vi "SETMODdll.vi"(8 "error in (no error)":errorcluster, 11 "Inputs":T2) -> (0 "error out":errorcluster, 3 "Outputs":T1)   [LabVIEW 2021]
doc: "subroutine SETMODdll(ncomp, htype, hmix, hcomp2, ierr, herr, htype_length, hmix_length, hcomp2_length, herr_length)\n\nSet model(s) other than the NIST-recommended (‘NBS’) ones.\n\nThis subroutine must be called before SETUP; it need not be called at all if the default (NIST-recommended)\nmodels are desired.\n\nINPUTS:\nncomp -- Number of components (1 for pure fluid) (integer)\nhtype -- Flag indicating which model to set (character*3)\n 'EOS': equation of state for thermodynamic properties\n 'ETA': viscosity\n 'TCX': thermal conductivity\n 'STN': surface tension\n 'NBS': reset all of the above model types and all subsidiary component models to 'NBS', values of hmix and hcomp are ignored.\nhmix -- Mixture model for the property specified in htype (character*3)\n Ignored if number of components = 1 \n Examples for hmix: \n ‘NBS’: use NIST recommendation for specified fluid/mixture \n ‘HMX’: mixture Helmholtz model for thermodynamic properties\n ‘ECS’: extended corresponding states for viscosity or therm. cond. \n ‘STX’: surface tension mixture model\nhcomp2 -- component model(s) to use for property specified in htype [array (1..ncomp) of character*3]\n 'NBS': NIST recommendation for specified fluid/mixture some allowable choices for an equation of state:\n 'FEQ': Helmholtz free energy model\n 'BWR': pure fluid modified Benedict-Webb-Rubin (MBWR)\n 'ECS': pure fluid thermo extended corresponding states some allowable choices for viscosity:\n 'ECS': extended corresponding states (all fluids)\n 'VS1': the 'composite' model for R134a, R152a, NH3, etc.\n 'VS2': Younglove-Ely model for hydrocarbons\n 'VS4': Generalized friction theory of Quinones-Cisneros and Deiters\n 'VS5': Chung et al. (1988) predictive model some allowable choices for thermal conductivity:\n 'ECS': extended corresponding states (all fluids)\n 'TC1': the 'composite' model for R134a, R152a, etc.\n 'TC2': Younglove-Ely model for hydrocarbons\n 'TC5': Chung et al. (1988) predictive model some allowable choices for surface tension:\n 'ST1': surface tension as f(tau); tau = 1 - T/Tc\n\nOUTPUTS:\nierr -- Error flag: 0 - Successful \n 113 - ncomp outside of bounds\nherr -- Error string (character*255)\nhtype_length -- length of variable htype (default: 3)\nhmix_length -- length of variable hmix (default: 3)\nhcomp2_length -- length of variable hcomp2 (default: 60)\nherr_length -- length of variable herr (default: 255)"
uses:
  REFPROP.dll
panel:
  # "REFPROP-SETMODdll.vi"
  # "void  SETMODdll(int32_t *ncomp, CStr htype, CStr hmix, CStr hcomp2, int32_t *ierr, CStr herr, int32_t htype_length, int32_t hmix_length, int32_t hcomp2_length, int32_t herr_length)"
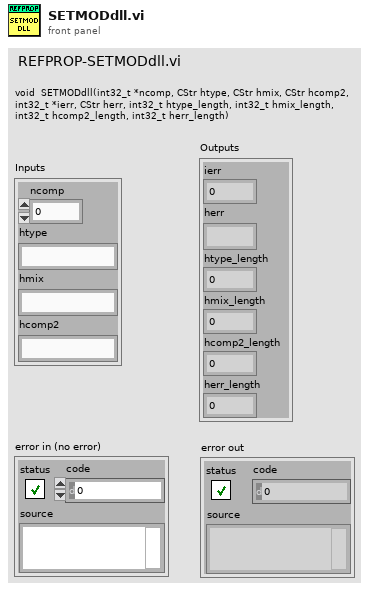
[diagram p1: front panel]
types:
  T1 = cluster{"ierr":i32, "herr":string, "htype_length":i32, "hmix_length":i32, "hcomp2_length":i32, "herr_length":i32}
  T2 = cluster{"ncomp":i32, "htype":string, "hmix":string, "hcomp2":string}
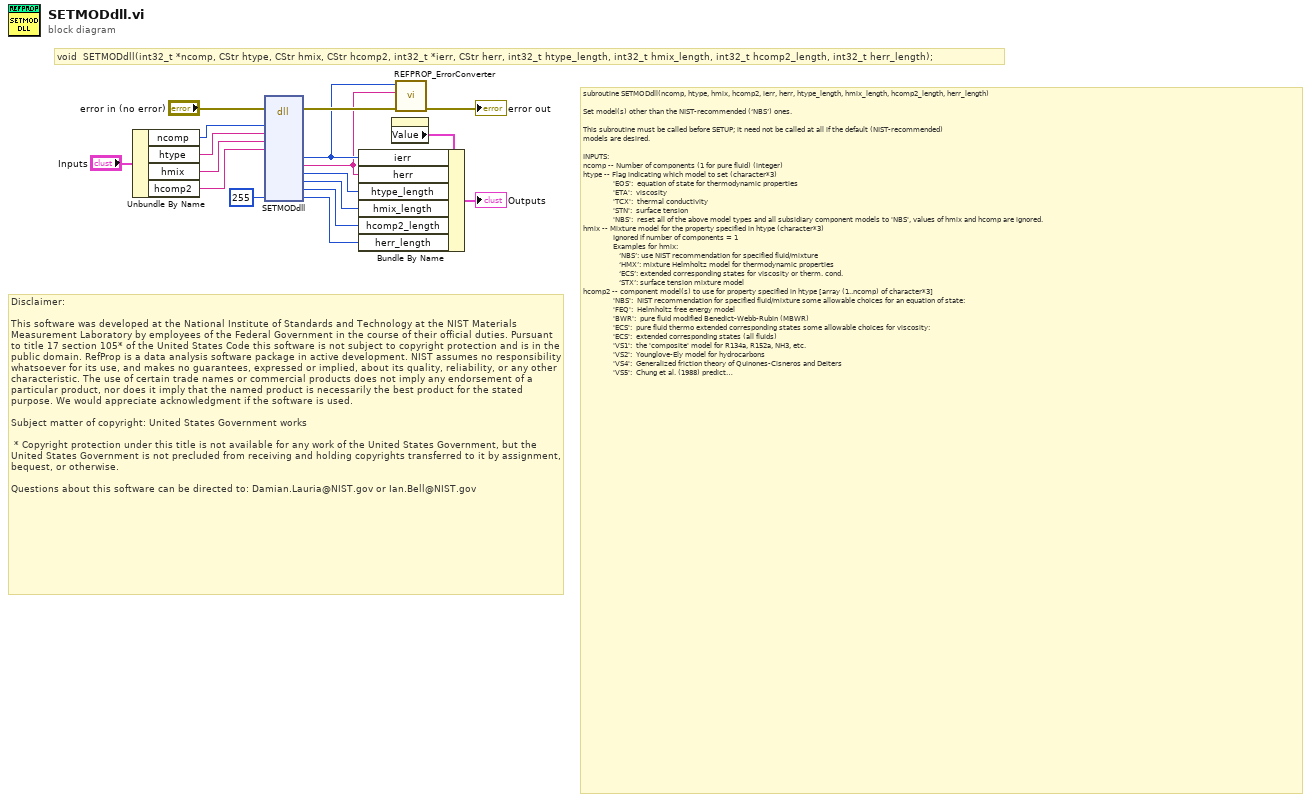
[diagram p0: block diagram]
diagram:
  # "Disclaimer:\n\nThis software was developed at the National Institute of Standards and Technology at the NIST Materials Measurement Laboratory by employees of the Federal Government in the course of their official duties. Pursuant to title 17 section 105* of the United States Code this software is not subject to copyright protection and is in the public domain. RefProp is a data analysis software package in active development. NIST assumes no responsibility whatsoever for its use, and makes no guarantees, expressed or implied, about its quality, reliability, or any other characteristic. The use of certain trade names or commercial products does not imply any endorsement of a particular product, nor does it imply that the named product is necessarily the best product for the stated purpose. We would appreciate acknowledgment if the software is used.\n \nSubject matter of copyright: United States Government works\n  \n * Copyright protection under this title is not available for any work of the United States Government, but the United States Government is not precluded from receiving and holding copyrights transferred to it by assignment, bequest, or otherwise.\n\nQuestions about this software can be directed to: Damian.Lauria@NIST.gov or Ian.Bell@NIST.gov"
  # "void  SETMODdll(int32_t *ncomp, CStr htype, CStr hmix, CStr hcomp2, int32_t *ierr, CStr herr, int32_t htype_length, int32_t hmix_length, int32_t hcomp2_length, int32_t herr_length);"
  # "subroutine SETMODdll(ncomp, htype, hmix, hcomp2, ierr, herr, htype_length, hmix_length, hcomp2_length, herr_length)\n\nSet model(s) other than the NIST-recommended (‘NBS’) ones.\n\nThis subroutine must be called before SETUP; it need not be called at all if the default (NIST-recommended)\nmodels are desired.\n\nINPUTS:\nncomp -- Number of components (1 for pure fluid) (integer)\nhtype -- Flag indicating which model to set (character*3)\n               'EOS':  equation of state for thermodynamic properties\n               'ETA':  viscosity\n               'TCX':  thermal conductivity\n               'STN':  surface tension\n               'NBS':  reset all of the above model types and all subsidiary component models to 'NBS', values of hmix and hcomp are ignored.\nhmix -- Mixture model for the property specified in htype (character*3)\n               Ignored if number of components = 1 \n               Examples for hmix: \n                  ‘NBS’: use NIST recommendation for specified fluid/mixture \n                  ‘HMX’: mixture Helmholtz model for thermodynamic properties\n                  ‘ECS’: extended corresponding states for viscosity or therm. cond. \n                  ‘STX’: surface tension mixture model\nhcomp2 -- component model(s) to use for property specified in htype [array (1..ncomp) of character*3]\n               'NBS':  NIST recommendation for specified fluid/mixture some allowable choices for an equation of state:\n               'FEQ':  Helmholtz free energy model\n               'BWR':  pure fluid modified Benedict-Webb-Rubin (MBWR)\n               'ECS':  pure fluid thermo extended corresponding states some allowable choices for viscosity:\n               'ECS':  extended corresponding states (all fluids)\n               'VS1':  the 'composite' model for R134a, R152a, NH3, etc.\n               'VS2':  Younglove-Ely model for hydrocarbons\n               'VS4':  Generalized friction theory of Quinones-Cisneros and Deiters\n               'VS5':  Chung et al. (1988) predictive model some allowable choices for thermal conductivity:\n               'ECS':  extended corresponding states (all fluids)\n               'TC1':  the 'composite' model for R134a, R152a, etc.\n               'TC2':  Younglove-Ely model for hydrocarbons\n               'TC5':  Chung et al. (1988) predictive model some allowable choices for surface tension:\n               'ST1':  surface tension as f(tau); tau = 1 - T/Tc\n\nOUTPUTS:\nierr -- Error flag: 0 - Successful \n                             113 - ncomp outside of bounds\nherr -- Error string (character*255)\nhtype_length -- length of variable htype (default: 3)\nhmix_length -- length of variable hmix (default: 3)\nhcomp2_length -- length of variable hcomp2 (default: 60)\nherr_length -- length of variable herr (default: 255)"
  n1 = Unbundle By Name("Inputs") -> ("ncomp"=w11:i32, "htype"=w10:string, "hmix"=w9:string, "hcomp2"=w8:string)
  n2 = dll-call lib="C:/Users/lauria/OneDrive - National Institute of Standards and Technology (NIST)/LabVIEW Projects/7 REFPROP/REFPROP-wrappers-master/REFPROP-wrappers-master/wrappers/Labview/REFPROP/REFPROP.*" fn="SETMODdll"(error in="error in (no error)", "ncomp"=w11, "htype"=w10, "hmix"=w9, "hcomp2"=w8, "herr_length"=255 ("ln4")) -> (error out=w16:errorcluster, "ierr"=w2:i32, "herr"=w1:string, "htype_length"=w6:i32, "hmix_length"=w5:i32, "hcomp2_length"=w4:i32, "herr_length"=w3:i32)  [unwired: 12 in, 1 out]
  n3 = property on="Outputs" class="Clust (strict)"() -> ("Value"=w7:T1)  [unwired: 2 in, 2 out]
  n4 = Bundle By Name(cluster=w7, "ierr"=w2, "herr"=w1, "htype_length"=w6, "hmix_length"=w5, "hcomp2_length"=w4, "herr_length"=w3) -> (→"Outputs":T1)
  n5 = call "REFPROP_ErrorConverter.vi"("error in (no error)"=w16, "Error Message"=w1, "Error Code"=w2) -> ("error out"=→"error out":errorcluster)  [unwired: 8 in]
